vi "epoll test.vi"() -> ()   [LabVIEW 2013]
uses:
  Source/C/Controls/epoll event struct.ctl
  Source/C/Controls/epoll events.ctl
  Source/C/Controls/epoll operations.ctl
  Source/Pipes/Classes/Unix Pipe/Unix Pipe.lvclass/Unix Pipe.ctl
  Source/Pipes/Classes/Unix Pipe Reader/Open Pipe (reader).vi
  Source/Pipes/Classes/Unix Pipe Writer/Open Pipe (writer).vi
  Source/Pipes/Classes/Unix Pipe Writer/Close Pipe (writer).vi
  Source/Pipes/Classes/Unix Pipe Reader/Close Pipe (reader).vi
  Source/C/Linux RT IPC.C.lvlib
  Source/Pipes/Linux RT IPC.Pipes.lvlib
  Source/Pipes/Classes/Unix Pipe Reader/Unix Pipe Reader.lvclass
  Source/Pipes/Classes/Unix Pipe/Unix Pipe.lvclass
  Source/Pipes/Classes/Unix Pipe Writer/Unix Pipe Writer.lvclass
panel:
  out "number of ready fds":i32
  out "Numeric":i32
  out "data":string
  in  "write":bool
  out "writer error out":errorcluster
  in  "stop":bool
  out "timed out":bool
  out "events":T1[](array[typedef])
  out "reader error out":errorcluster
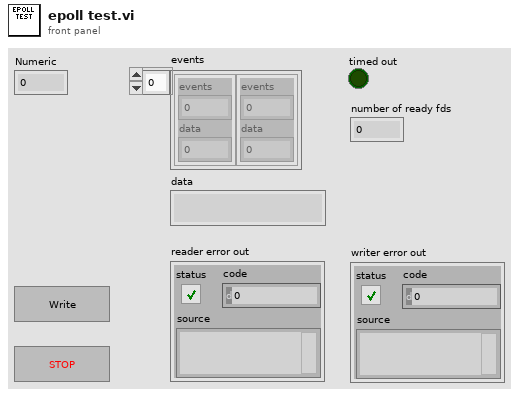
[diagram p1: front panel]
types:
  T1 = typedef "Linux RT IPC.C.lvlib/epoll event struct.ctl" = cluster{"events":u32, "data":u64}
  T2 = typedef "Linux RT IPC.C.lvlib/epoll operations.ctl" = u32
  T3 = typedef "Linux RT IPC.C.lvlib/epoll events.ctl" = u32
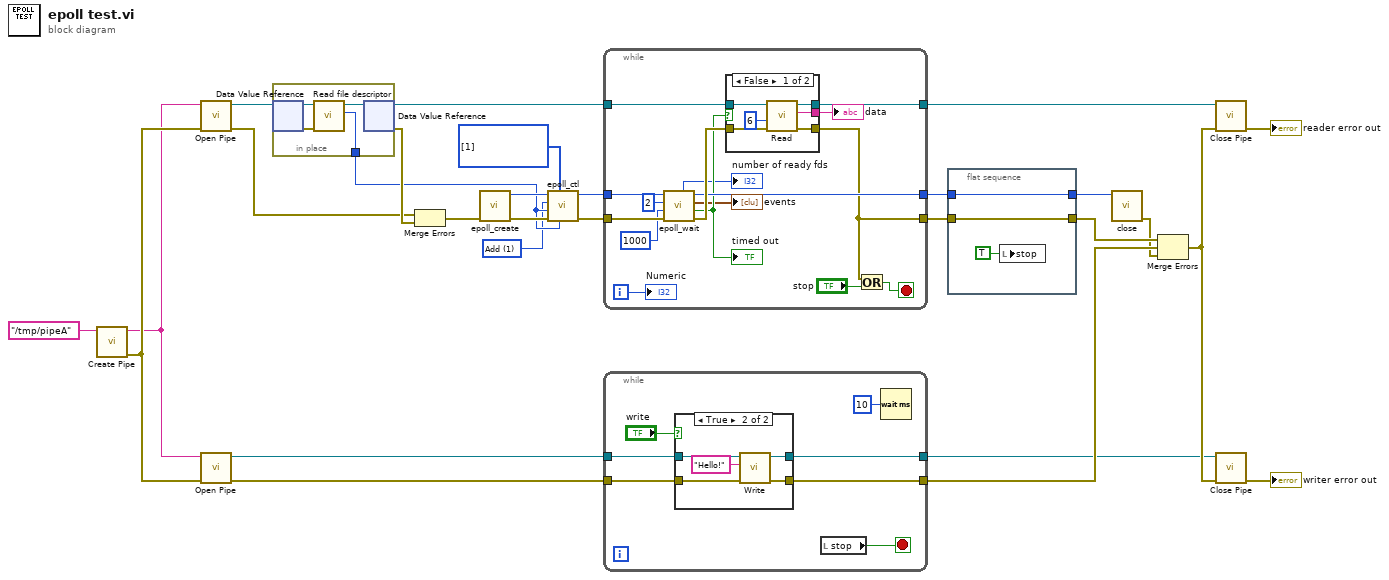
[diagram p0: block diagram]
diagram:
  w1 = T2 1 items=["Add"=1, "Delete"=2, "Modify"=3] ("operation")
  w22 = T3[] [1] items=["EPOLLIN"=1, "EPOLLPRI"=2, "EPOLLOUT"=4, "EPOLLERR"=8, "EPOLLHUP"=16, "EPOLLRDNORM"=64, "EPOLLRDBAND"=128, "EPOLLWRNORM"=256, "EPOLLWRBAND"=512, "EPOLLMSG"=1024, "EPOLLRDHUP"=8192, "EPOLLWAKEUP"=536870912, "EPOLLONESHOT"=1073741824, "EPOLLET"=2147483648] ("epoll events (default: none)")
  n1 = call "Create Pipe.vi"("pathname in"="/tmp/pipeA") -> ("error out"=w7:errorcluster, "pathname out"=w6:string)  [unwired: 8 in, 1 out]
  n2 = call-poly "Open Pipe.vi"("error in (no error)"=w7, "pathname in"=w6) -> ("error out"=w26:errorcluster, "pipe reader out"=w28:refnum<data-value>)  [unwired: 8 in]
  n3 = call-poly "Open Pipe.vi"("error in (no error)"=w7, "pathname in"=w6) -> ("error out"=w13:errorcluster, "pipe writer out"=w14:refnum<data-value>)  [unwired: 8 in]
  n4 = in-place {
    in-place-border: [w29] -> w21
    n5 = in-place-dvr #1(w28) -> (w32:refnum<class "Unix Pipe Reader.lvclass">, w30:errorcluster)
    n6 = call "Read file descriptor.vi"("error in (no error)"=w30, "Unix Pipe in"=w32) -> ("file descriptor"=w29:i32, "Unix Pipe out"=w31:refnum<class "Unix Pipe Reader.lvclass">)  [unwired: 7 in, 1 out]
    n7 = in-place-dvr #1(w31) -> (w16:refnum<data-value>, w27:errorcluster)
  }
  n8 = Merge Errors(w26, w27) -> (w25:errorcluster)
  n9 = call "epoll_create.vi"("error in (no error)"=w25) -> ("error out"=w24:errorcluster, "epfd"=w23:i32)  [unwired: 9 in]
  n10 = call "epoll_ctl.vi"("epoll data"=w21, "epoll events (default: none)"=w22, "error in (no error)"=w24, "target fd"=w21, "operation"=w1, "epfd in"=w23) -> ("error out"=w20:errorcluster, "epfd out"=w19:i32)  [unwired: 4 in]
  n11 = while {
    tunnel: w20 -> [w47]
    tunnel: w19 -> [w46]
    tunnel: [w45] -> w11
    tunnel: [w38] -> w12
    tunnel: w16 -> [w43]
    tunnel: [w42] -> w15
    i -> [w35]
    stop <- w39 stop-if-true
    n12 = call "epoll_wait.vi"("error in (no error)"=w47, "timeout ms (-1)"=1000 ("timeout ms (10)"), "max events"=u32 2, "epfd in"=w46) -> ("error out"=w48:errorcluster, "timed out"=w36:bool, "events"=→"events":T1[], "epfd out"=w45:i32, "number of ready fds"=→"number of ready fds":i32)  [unwired: 3 in]
    "timed out" <- w36
    n13 = case shown="False" w36 {
      tunnel: w48 -> [w49 w56]
      tunnel: w43 -> [w54 w55]
      tunnel: [w53 w55] -> w42
      tunnel: [w52 _] -> w41
      tunnel: [w50 w56] -> w38
      frame False {
        n14 = call "Read.vi"("error in (no error)"=w49, "bytes to read"=6, "pipe reader in"=w54) -> ("error out"=w50:errorcluster, "data"=w52:string, "pipe reader out"=w53:refnum<data-value>)  [unwired: 4 in, 2 out]
      }
      frame True {
      }
    }
    "data" <- w41
    n15 = Or(x=w38, y="stop") -> (x .or. y?=w39:bool)
    "Numeric" <- w35
  }
  n16 = while {
    tunnel: w14 -> [w62]
    tunnel: w13 -> [w61]
    tunnel: [w59] -> w2
    tunnel: [w58] -> w5
    stop <- w60 stop-if-true
    n17 = case shown="True" "write" {
      tunnel: w62 -> [w65 w70]
      tunnel: w61 -> [w64 w69]
      tunnel: [w65 w68] -> w59
      tunnel: [w64 w67] -> w58
      frame False {
      }
      frame True {
        n18 = call "Write.vi"("error in (no error)"=w69, "data"="Hello!", "pipe writer in"=w70) -> ("error out"=w67:errorcluster, "pipe writer out"=w68:refnum<data-value>)  [unwired: 6 in, 1 out]
      }
    }
    n19 = local read "stop"() -> (w60:bool)
    n20 = Wait (ms)(milliseconds to wait=u32 10) -> ()  [unwired: 1 out]
  }
  n21 = flat-sequence {
    tunnel: w12 -> [w73]
    tunnel: w11 -> [w72]
    tunnel: [w73] -> w10
    tunnel: [w72] -> w9
    frame #0 {
      n22 = local write "stop"(TRUE ("stop")) -> ()
    }
  }
  n23 = call "close.vi"("file descriptor in"=w9) -> ("error out"=w4:errorcluster)  [unwired: 10 in]
  n24 = Merge Errors(w10, w5, w4) -> (w3:errorcluster)
  n25 = call-poly "Close Pipe.vi"("error in (no error)"=w3, "pipe in"=w15) -> ("error out"=→"reader error out":errorcluster)  [unwired: 8 in, 1 out]
  n26 = call-poly "Close Pipe.vi"("error in (no error)"=w3, "pipe in"=w2) -> ("error out"=→"writer error out":errorcluster)  [unwired: 8 in, 1 out]
